vi "Image_Folder_2.0.vi"(8 "New":i32, 9 "Old":i32, 10 "Other":i32, 11 "Data":T1={"Camera 1"={"Camera1"="", "Cam 1"=FALSE, "CAM1 Model"=enum."a2A5328-15ucBAS", "Cam1 ID"=0}, "Camera 2"={"Camera2"="", "Cam 2"=FALSE, "CAM2 Model"=enum."a2A5328-15ucBAS", "Cam2 ID"=0}, "Image"={"Camera1_Img"=refnum, "Camera2_Img"=refnum, "Img1_Orig_Disp"=refnum, "Img2_Orig_Disp"=refnum, "Img1_Orig_RGB"=refnum, "Img2_Orig_RGB"=refnum, "Blue_Plane_Extract"=refnum, "Subtracted_Plane"=refnum, "Img1_Binary"=refnum, "Img2_Binary"=refnum, "Crop_Mask"=refnum, "Img1_Save"=refnum, "Img2_Save"=refnum, "Img1_Cali_Full"=refnum, "Img2_Cali_Full"=refnum, "Img1_Cali_Detect"=refnum, "Img2_Cali_Detect"=refnum}, "Ques"={"Cam 1 queue"=refnum, "Cam 2 queue"=refnum, "Cam 1 - save queue"=refnum, "Cam 2 - save queue"=refnum, "Image Process Queue Size"=500, "Image Save Queue Size"=500, "Overload threshold"=500, "Max large object threshold"=0}, "Arduino SRS"={"Pinch-valve"="", "Actuator"=FALSE, "Open(T)/Close(F)"=FALSE, "Arduino Uno"=""}, "Pump"={"Port"="", "Connection"=FALSE, "Flush Size"=0, "Command"="", "Pump Size"=enum."Large", "Pump"=""}, "Camera settings"={"Detection settings"={"Sample size threshold"=500, "Detection Region %"=30.0, "Timeout Sample"=200}, "Lens/camera settings"={"Aperture"=enum."Item 0", "Legacy Cam Attributes"=FALSE, "Max Framerate"=100, "Exposure Time"=1000.0, "Framerate"=15}, "Crop settings"={"Cam1"={"Rectangle 1"={"Left"=0, "Top"=0, "Right"=0, "Bottom"=0, "Rotation"=0.0}, "Camera Orientation 1"="", "Pixel to mm 1"=0.0}, "Cam2"={"Rectangle 2"={"Left"=0, "Top"=0, "Right"=0, "Bottom"=0, "Rotation"=0.0}, "Camera Orientation 2"="", "Pixel to mm 2"=0.0}}}, "Arduino ISS"={"Mega F3"="", "Phase3"=FALSE, "Barcode"="", "Sorting sys."=FALSE, "Initial size"=0.0, "Size Interval"=0.0, "Mun. of containers"=0.0, "Container nr."=0.0, "Arduino Mega"=""}, "Img_Capt"=FALSE, "Empty_Refill"=FALSE, "I don't think is in use"={"Light intensity"=100}, "Extended setup"={"Location"="Station", "Latitude"="Station", "Longitude"="Station", "Determiner"="Station", "Sex"="Station", "Station"="", "Collection date"=""}, "Main interface"={"Sample Name"="Test Sample", "Operator"="JFR", "Species Name"="", "Other Notes"=""}, "Tap1"=0, "SystemVersion"=0, "System Serial"="", "Exit"=FALSE, "Kuvette Full"=FALSE, "Core JKI"={"Current VI Reference"=refnum, "Close Panel on Exit?"=FALSE}, "Calibration"={"Calibration 1"=path "C:/Users/au540322/Desktop/IHS_Project/images/Debris/Debris_0/Debris_0_2019_06_01-23-32-49-686.PNG", "Calibration 2"=path "C:/Users/au540322/Desktop/IHS_Project/images/Debris/Debris_0/Debris_0_2019_06_01-23-32-49-686.PNG", "Detect 1"=path "C:/Users/au540322/Desktop/IHS_Project/images/Debris/Debris_0/Debris_0_2019_06_01-23-32-49-686.PNG", "Detect 2"=path "C:/Users/au540322/Desktop/IHS_Project/images/Debris/Debris_0/Debris_0_2019_06_01-23-32-49-686.PNG"}, "Flush Insect"=FALSE, "Auto Flush"=FALSE} {"SystemVersion" items=["Standard", "XL"]; "Tap1" items=["Session Data", "Extended Setup", "Buffer", "Camera", "Dispenser", "Stats", "Connections"]; "I don't think is in use"."Light intensity" scale=0.0..100.0; "Camera settings"."Crop settings"."Cam2"."Rectangle 2"."Rotation" format="%.2f"; "Camera settings"."Crop settings"."Cam2"."Rectangle 2"."Left" scale=0.0..1024.0; "Camera settings"."Crop settings"."Cam2"."Rectangle 2"."Right" scale=0.0..1024.0; "Camera settings"."Crop settings"."Cam1"."Rectangle 1"."Rotation" format="%.2f"; "Camera settings"."Crop settings"."Cam1"."Rectangle 1"."Left" scale=0.0..1024.0; "Camera settings"."Crop settings"."Cam1"."Rectangle 1"."Right" scale=0.0..1024.0; "Camera settings"."Lens/camera settings"."Framerate" min=1; "Camera settings"."Lens/camera settings"."Max Framerate" min=1; "Camera settings"."Detection settings"."Sample size threshold" min=1; "Pump"."Flush Size" min=0 max=6000 step=100; "Ques"."Overload threshold" min=1; "Ques"."Image Save Queue Size" min=1; "Ques"."Image Process Queue Size" min=1}) -> (2 "Subfolder Name":string, 3 "Subfolder Path":string)   [LabVIEW 2024]
uses:
  controls/Data_JKI.ctl
  <vilib>/userDefined/High Color/IMAQdx.ctl
  <vilib>/vision/Image Controls.llb/IMAQ Image.ctl
panel:
  out "error out 2":errorcluster
  out "error out":errorcluster
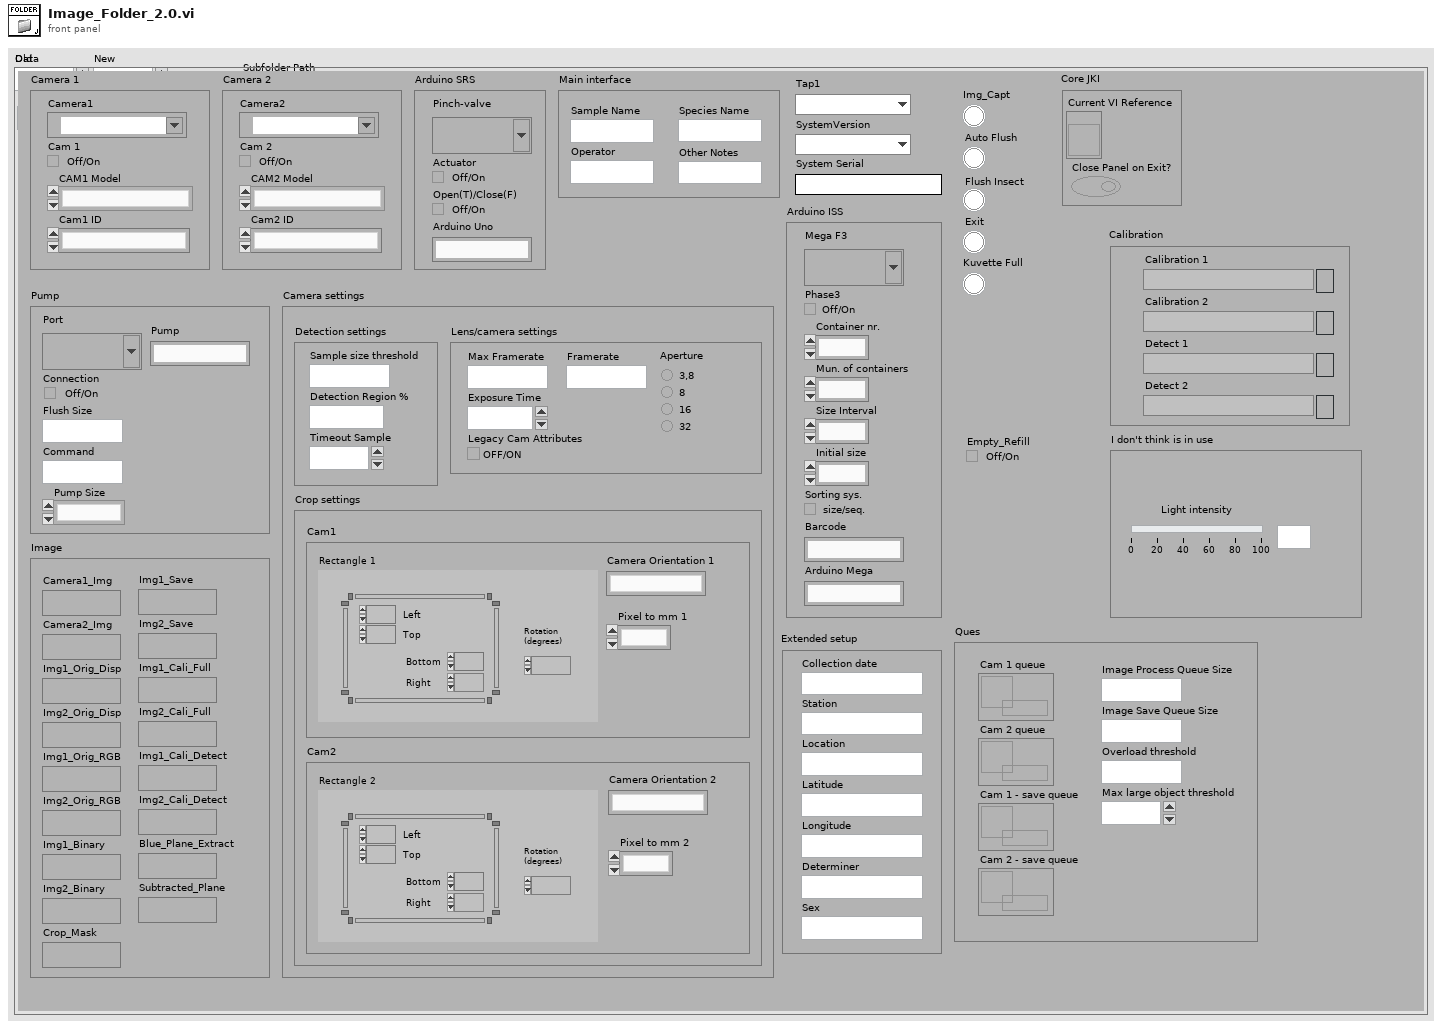
[diagram p1: front panel]
types:
  T1 = typedef "Data_JKI.ctl" = cluster{"Camera 1":cluster{"Camera1":T2, "Cam 1":bool, "CAM1 Model":enum16{"a2A5328-15ucBAS", "acA1920-155uc"}, "Cam1 ID":i32}, "Camera 2":cluster{"Camera2":T2, "Cam 2":bool, "CAM2 Model":enum16{"a2A5328-15ucBAS", "acA1920-155uc"}, "Cam2 ID":i32}, "Image":cluster{"Camera1_Img":T3, "Camera2_Img":T3, "Img1_Orig_Disp":T3, "Img2_Orig_Disp":T3, "Img1_Orig_RGB":T3, "Img2_Orig_RGB":T3, "Blue_Plane_Extract":T3, "Subtracted_Plane":T3, "Img1_Binary":T3, "Img2_Binary":T3, "Crop_Mask":T3, "Img1_Save":T3, "Img2_Save":T3, "Img1_Cali_Full":T3, "Img2_Cali_Full":T3, "Img1_Cali_Detect":T3, "Img2_Cali_Detect":T3}, "Ques":cluster{"Cam 1 queue":refnum<queue>, "Cam 2 queue":refnum<queue>, "Cam 1 - save queue":refnum<queue>, "Cam 2 - save queue":refnum<queue>, "Image Process Queue Size":i32, "Image Save Queue Size":i32, "Overload threshold":i32, "Max large object threshold":i32}, "Arduino SRS":cluster{"Pinch-valve":refnum<visa-resource-name>, "Actuator":bool, "Open(T)/Close(F)":bool, "Arduino Uno":string}, "Pump":cluster{"Port":refnum<visa-resource-name>, "Connection":bool, "Flush Size":i32, "Command":string, "Pump Size":enum16{"None", "Small", "Large"}, "Pump":string}, "Camera settings":cluster{"Detection settings":cluster{"Sample size threshold":i32, "Detection Region %":dbl, "Timeout Sample":i32}, "Lens/camera settings":cluster{"Aperture":enum32{"Item 0", "Item 1", "Item 2", "Item 3"}, "Legacy Cam Attributes":bool, "Max Framerate":i32, "Exposure Time":dbl, "Framerate":i32}, "Crop settings":cluster{"Cam1":cluster{"Rectangle 1":T4, "Camera Orientation 1":string, "Pixel to mm 1":dbl}, "Cam2":cluster{"Rectangle 2":T4, "Camera Orientation 2":string, "Pixel to mm 2":dbl}}}, "Arduino ISS":cluster{"Mega F3":refnum<visa-resource-name>, "Phase3":bool, "Barcode":string, "Sorting sys.":bool, "Initial size":dbl, "Size Interval":dbl, "Mun. of containers":dbl, "Container nr.":dbl, "Arduino Mega":string}, "Img_Capt":bool, "Empty_Refill":bool, "I don't think is in use":cluster{"Light intensity":i32}, "Extended setup":cluster{"Location":string, "Latitude":string, "Longitude":string, "Determiner":string, "Sex":string, "Station":string, "Collection date":string}, "Main interface":cluster{"Sample Name":string, "Operator":string, "Species Name":string, "Other Notes":string}, "Tap1":u16, "SystemVersion":u16, "System Serial":string, "Exit":bool, "Kuvette Full":bool, "Core JKI":cluster{"Current VI Reference":refnum<vi>, "Close Panel on Exit?":bool}, "Calibration":cluster{"Calibration 1":path, "Calibration 2":path, "Detect 1":path, "Detect 2":path}, "Flush Insect":bool, "Auto Flush":bool}
  T2 = typedef "IMAQdx.ctl" = refnum<k21>
  T3 = typedef "IMAQ Image.ctl" = refnum<image>
  T4 = typedef "IMAQ Rectangle" = cluster{"Left":i32, "Top":i32, "Right":i32, "Bottom":i32, "Rotation":dbl}
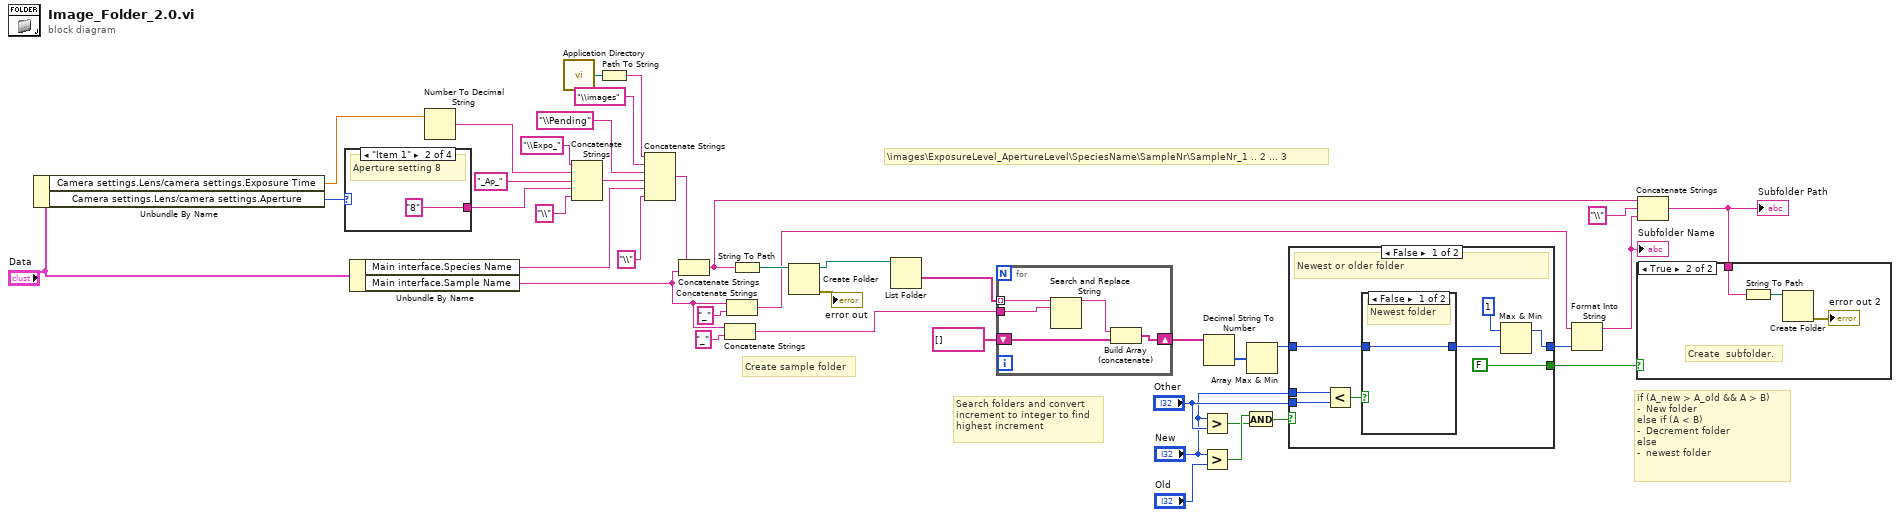
[diagram p0: block diagram]
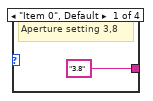
[diagram p2: hidden frame]
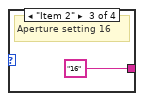
[diagram p3: hidden frame]
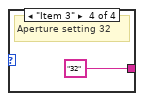
[diagram p4: hidden frame]
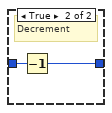
[diagram p5: hidden frame]
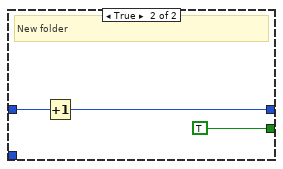
[diagram p6: hidden frame]
diagram:
  # "\\images\\ExposureLevel_ApertureLevel\\SpeciesName\\SampleNr\\SampleNr_1 .. 2 ... 3"
  # "if (A_new > A_old && A > B)\n-  New folder\nelse if (A < B)\n-  Decrement folder\nelse \n-  newest folder"
  # "Search folders and convert \nincrement to integer to find\nhighest increment"
  # "Create sample folder"
  n1 = Unbundle By Name("Data") -> ("Camera settings.Lens/camera settings.Exposure Time"=w13:dbl, "Camera settings.Lens/camera settings.Aperture"=w10:enum32{"Item 0", "Item 1", "Item 2", "Item 3"})
  n2 = case shown="\"Item 1\"" w10 {
    tunnel: ["3.8" "8" "16" "32"] -> w8
    frame "Item 0", Default {
      # "Aperture setting 3,8"
    }
    frame "Item 1" {
      # "Aperture setting 8"
    }
    frame "Item 2" {
      # "Aperture setting 16"
    }
    frame "Item 3" {
      # "Aperture setting 32"
    }
  }
  n3 = Unbundle By Name("Data") -> ("Main interface.Species Name"=w18:string, "Main interface.Sample Name"=w16:string)
  n4 = Number To Decimal String(number=w13) -> (decimal integer string=w9:string)  [unwired: 1 in]
  n5 = call <vilib>:"Application Directory.vi"() -> ("Application Directory"=w36:path)
  n6 = Concatenate Strings("\\Expo_" ("string"), w9, "_Ap_" ("string"), w8, "\\" ("string")) -> (w6:string)
  n7 = Path To String(path=w36) -> (string=w4:string)
  n8 = Concatenate Strings(w4, "\\images" ("string"), "\\Pending" ("string"), w6, w18, "\\" ("string")) -> (w17:string)
  n9 = Concatenate Strings(w17, w16) -> (w15:string)
  n10 = Concatenate Strings(w16, "_" ("string")) -> (w34:string)
  n11 = Concatenate Strings(w16, "_" ("string")) -> (w5:string)
  n12 = String To Path(string=w15) -> (path=w37:path)
  n13 = Create Folder(path (use dialog)=w37) -> (created path=w40:path, error out=→"error out":errorcluster)  [unwired: 2 in, 1 out]
  n14 = List Folder(path=w40) -> (folder names=w35:string[])  [unwired: 3 in, 3 out]
  n15 = for {
    tunnel: w35 -> [w50] mode=indexing
    tunnel: w34 -> [w49]
    shift-right: [w47] -> w32
    shift-left: string[] [] -> [w46]
    n16 = Search and Replace String(input string=w50, search string=w49) -> (result string=w48:string)  [unwired: 6 in, 3 out]
    n17 = Build Array (concatenate)(w48, w46) -> (w47:string[])
  }
  n18 = Greater?(x="New", y="Other") -> (0:w26:bool)
  n19 = Greater?(x="New", y="Old") -> (0:w27:bool)
  n20 = Decimal String To Number(string=w32) -> (number=w31:i32[])  [unwired: 2 in, 1 out]
  n21 = And(x=w27, y=w26) -> (x .and. y?=w25:bool)
  n22 = Array Max & Min(array=w31) -> (max value=w21:i32)  [unwired: 3 out]
  n23 = case shown="False" w25 {
    tunnel: "Other" -> [w58 _]
    tunnel: "New" -> [w57 _]
    tunnel: [FALSE ("New sample (F)") TRUE ("New sample (F)")] -> w22
    tunnel: w21 -> [w55 w63]
    tunnel: [w51 w62] -> w20
    frame False {
      # "Newest or older folder"
      n24 = Less?(x=w57, y=w58) -> (x < y?=w56:bool)
      n25 = case shown="False" w56 {
        tunnel: w55 -> [w59 w61]
        tunnel: [w59 w60] -> w53
        frame False {
          # "Newest folder"
        }
        frame True {
          # "Decrement"
          n26 = Decrement(x=w61) -> (x-1=w60:i32)
        }
      }
      n27 = Max & Min(x=1, y=w53) -> (max(x,y)=w51:i32)  [unwired: 1 out]
    }
    frame True {
      # "New folder"
      n28 = Increment(x=w63) -> (x+1=w62:i32)
    }
  }
  n29 = Format Into String(initial string=w5, w20) -> (resulting string=w29:string)  [unwired: 2 in, 1 out]
  "Subfolder Name" <- w29
  n30 = Concatenate Strings(w15, "\\" ("string"), w29) -> (w19:string)
  "Subfolder Path" <- w19
  n31 = case shown="True" w22 {
    tunnel: w19 -> [_ w65]
    frame False {
    }
    frame True {
      # "Create  subfolder."
      n32 = String To Path(string=w65) -> (path=w66:path)
      n33 = Create Folder(path (use dialog)=w66) -> (error out=→"error out 2":errorcluster)  [unwired: 2 in, 2 out]
    }
  }
